vi "Escribir_propiedades_2.vi"() -> ()   [LabVIEW 2016]
panel:
  in  "Stop Button":bool
  out "Boolean":bool
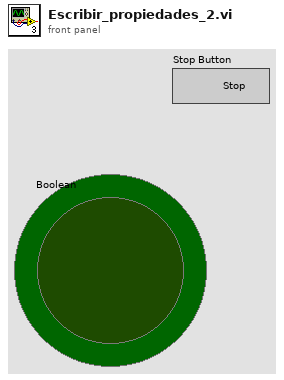
[diagram p1: front panel]
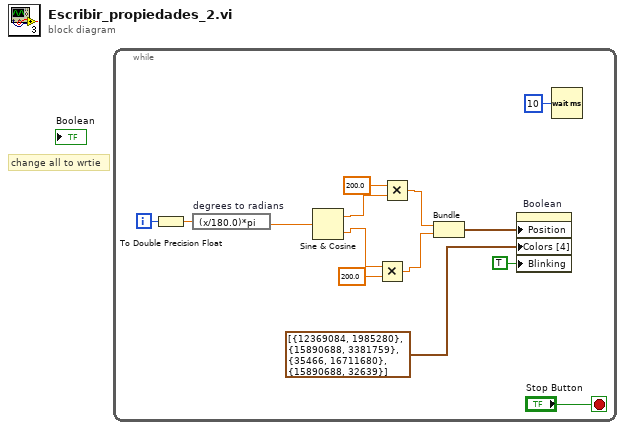
[diagram p0: block diagram]
diagram:
  # "change all to wrtie"
  n1 = while {
    i -> [w12]
    stop <- "Stop Button" stop-if-true
    n2 = To Double Precision Float(number=w12) -> (double precision float=w11:dbl)
    n3 = expression code="(x/180.0)*pi" "degrees to radians"(w11) -> (w10:dbl)
    n4 = Sine & Cosine(0:w10) -> (1:w9:dbl, 2:w8:dbl)
    n5 = Multiply(x=w8, y=200.0) -> (x*y=w4:dbl)
    n6 = Multiply(x=200.0, y=w9) -> (x*y=w5:dbl)
    n7 = Bundle(w5, w4) -> (w3:cluster{dbl, dbl})  [unwired: 1 in]
    n8 = property on="Boolean" class="Bool (strict)"("Position"=w3, "Colors [4]"=cluster{u32, u32}[] [{12369084, 1985280}, {15890688, 3381759}, {35466, 16711680}, {15890688, 32639}], "Blinking"=TRUE) -> ()  [unwired: 2 in, 2 out]
    n9 = Wait (ms)(milliseconds to wait=u32 10) -> ()  [unwired: 1 out]
  }
